vi "Autonomous Independent.vi"   [LabVIEW 2012]
doc: "This VI is called when autonomous begins, and will automatically be terminated when autonomous ends. You can carry out timed or sensor driven robot movement independently without needing to return to the caller."
uses:
  <vilib>/Rock Robotics/WPI/DriverStation/DriverStationLCD/WPI_DriverStationLCDLCDLine.ctl
  Begin/Global Variables.vi
panel:
  # "Be sure to right-click and choose Data Operations>>Make Current Value default if you want to save the array values with the VI"
types:
  T1 = typedef "WPI_DriverStationLCDLCDLine.ctl" = enum16{"Main - Line 1", "User - Line 2", "User - Line 3", "User - Line 4", "User - Line 5", "User - Line 6"}
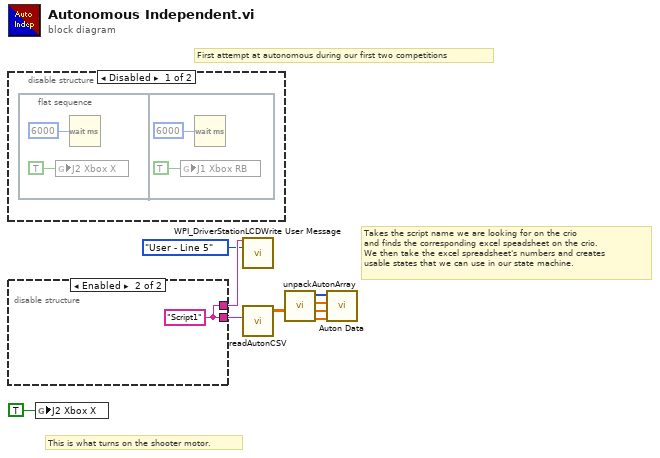
[diagram p0: block diagram]
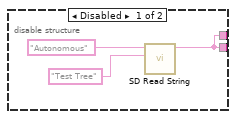
[diagram p2: hidden frame]
diagram:
  # "This is what turns on the shooter motor."
  # "Takes the script name we are looking for on the crio\nand finds the corresponding excel speadsheet on the crio.\nWe then take the excel spreadsheet's numbers and creates\nusable states that we can use in our state machine."
  # "First attempt at autonomous during our first two competitions"
  n1 = disable-structure shown="Disabled" {
    frame Disabled {
      n2 = flat-sequence {
        frame #0 {
          n3 = global write "Global Variables.vi" "J2 Xbox X"(TRUE) -> ()
          n4 = Wait (ms)(milliseconds to wait=u32 6000) -> ()  [unwired: 1 out]
        }
        frame #1 {
          n5 = global write "Global Variables.vi" "J1 Xbox RB"(TRUE ("Shoot trigger")) -> ()
          n6 = Wait (ms)(milliseconds to wait=u32 6000) -> ()  [unwired: 1 out]
        }
      }
    }
    frame Enabled {
    }
  }
  n7 = disable-structure shown="Enabled" {
    disable-tunnel: [w15 w17] -> w9
    disable-tunnel: [w15 w17] -> w2
    frame Disabled {
      n8 = call <vilib>:"SD Read String.vi"("Table Prefix"="Test Tree", "Name"="Autonomous") -> ("String"=w15:string)  [unwired: 7 in, 2 out]
    }
    frame Enabled {
      w17 = "Script1" ("AutonFile")
    }
  }
  n9 = global write "Global Variables.vi" "J2 Xbox X"(TRUE) -> ()
  n10 = call <vilib>:"WPI_DriverStationLCDWrite User Message.vi"("line text"=w2, "line"=WPI_DriverStationLCDLCDLine."User - Line 5") -> ()  [unwired: 13 in, 1 out]
  n11 = call "readAutonCSV.vi"("AutonFile"=w9) -> ("AutonArray"=w8:dbl[][])  [unwired: 7 in]
  n12 = call "unpackAutonArray.vi"("all rows"=w8) -> ("Power"=w3:dbl[], "Distance/Time"=w4:dbl[], "Heading"=w5:dbl[], "Primitive"=w6:i16[])  [unwired: 6 in, 1 out]
  n13 = call "Auton Data.vi"("power"=w3, "time/distance"=w4, "Heading"=w5, "primitive ID"=w6) -> ()  [unwired: 8 in]
